vi "FPGA Calibration.vi"(8 "error in":errorcluster, 11 "FPGA Interface":T1) -> (0 "error out":errorcluster, 3 "FPGA Interface 2":T1)   [LabVIEW 2015]
uses:
  Formula Hybrid 2012 r1/FPGA Typedef.ctl
  <vilib>/rvi/errors/niLvFpgaAdjustHostInterfaceError.vi
  <vilib>/Utility/error.llb/Error Cluster From Error Code.vi
  <vilib>/rvi/interface/nirviReadWriteControl/nirviReadWriteControl.xnode
  FPGA Bitfiles/Latest.lvbitx
  NiFpgaLv.dll
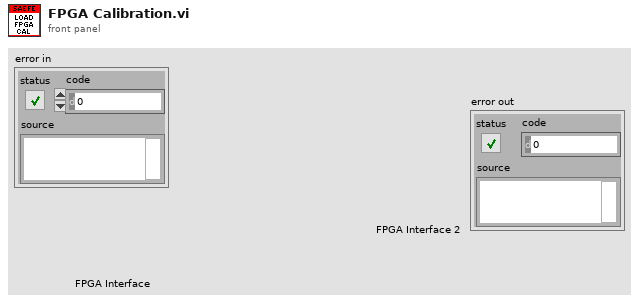
[diagram p1: front panel]
types:
  T1 = typedef "FPGA Typedef.ctl" = refnum<k20>
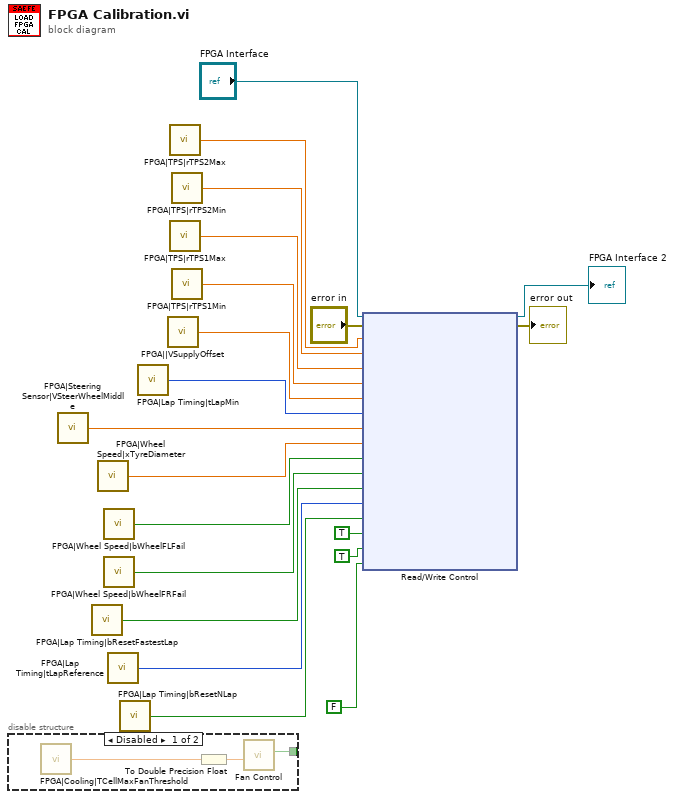
[diagram p0: block diagram]
diagram:
  n1 = disable-structure shown="Disabled" {
    disable-tunnel: [w23 _] -> _
    frame Disabled {
      n2 = call "FPGA|Cooling|TCellMaxFanThreshold"() -> ("Value"=w22:sgl)
      n3 = To Double Precision Float(number=w22) -> (double precision float=w21:dbl)
      n4 = call "Fan Control.vi"("TCellFanStart"=w21) -> ("PWM Out"=w23:bool)  [unwired: 9 in, 1 out]
    }
    frame Enabled {
    }
  }
  n5 = call "FPGA|Steering Sensor|VSteerWheelMiddle"() -> ("Value"=w12:sgl)
  n6 = call "FPGA|Lap Timing|bResetFastestLap"() -> ("Value"=w8:bool)
  n7 = call "FPGA|Wheel Speed|xTyreDiameter"() -> ("Value"=w11:sgl)
  n8 = call "FPGA|Wheel Speed|bWheelFLFail"() -> ("Value"=w10:bool)
  n9 = call "FPGA|Wheel Speed|bWheelFRFail"() -> ("Value"=w9:bool)
  n10 = call "FPGA|Lap Timing|tLapReference"() -> ("Value"=w7:u32)
  n11 = call "FPGA|Lap Timing|bResetNLap"() -> ("Value"=w6:bool)
  n12 = call "FPGA|Lap Timing|tLapMin"() -> ("Value"=w13:u32)
  n13 = call "FPGA||VSupplyOffset"() -> ("Value"=w14:sgl)
  n14 = call "FPGA|TPS|rTPS2Max"() -> ("Value"=w18:sgl)
  n15 = call "FPGA|TPS|rTPS1Max"() -> ("Value"=w16:sgl)
  n16 = call "FPGA|TPS|rTPS2Min"() -> ("Value"=w17:sgl)
  n17 = call "FPGA|TPS|rTPS1Min"() -> ("Value"=w15:sgl)
  n18 = xnode "Read/Write Control"("FPGA VI Reference In"="FPGA Interface", "error in"="error in", "rTPS2Max"=w18, "rTPS2Min"=w17, "rTPS1Max"=w16, "rTPS1Min"=w15, "VSupplyOffset"=w14, "tLapMin"=w13, "VSteerWheelMiddle"=w12, "Tire Diameter(m)"=w11, "bWheelFLFail"=w10, "bWheelFRFail"=w9, "bResetFastestLap"=w8, "tLapReference"=w7, "bResetNLap"=w6, "bLapBeaconPickupEnable"=TRUE, "bWheelSpeedsEnable"=TRUE, "bAccumulatorFansEnable"=FALSE) -> ("FPGA VI Reference Out"=→"FPGA Interface 2":T1, "error out"=→"error out":errorcluster)
